vi "nPoints Concept - Servo Motor.vi"() -> ()   [LabVIEW 2014]
uses:
  <vilib>/myRIO/Express VI/Onboard IO/PWM/PWM Express VI.xnode
  <vilib>/myRIO/Instrument Drivers/Onboard IO/PWM/vis/Set Duty Cycle and Frequency.vi
  <vilib>/myRIO/Instrument Drivers/Onboard IO/PWM/PWM.lvlib
  <vilib>/myRIO/Instrument Drivers/Onboard IO/PWM/typedefs/PWM Configuration.ctl
  <vilib>/myRIO/Common/Instrument Driver Framework/myRIO v1.0/PWM/typedefs/PWM Channels Enum.ctl
  <vilib>/myRIO/Common/Instrument Driver Framework/Utilities/typedefs/Generic FPGA Reference.ctl
  <vilib>/myRIO/Common/Instrument Driver Framework/Utilities/typedefs/myRIO v1.0 Reference.ctl
  <vilib>/myRIO/Common/Instrument Driver Framework/Utilities/typedefs/Hardware Version Enum.ctl
  <vilib>/myRIO/Common/Instrument Driver Framework/Utilities/typedefs/myRIO Generic Hardware Reference.ctl
  <vilib>/myRIO/Instrument Drivers/Onboard IO/PWM/typedefs/PWM Reference.ctl
  <vilib>/myRIO/Instrument Drivers/Onboard IO/PWM/vis/myRIO PWM Open.xnode
  <vilib>/myRIO/Common/Instrument Driver Framework/Utilities/vis/Is FPGA Ref Available.vi
  <vilib>/myRIO/Common/Instrument Driver Framework/myRIO v1.0/PWM/vis/myRIO v1.1 Open PWM.vi
  <vilib>/userdefined/High Color/nirio_resource_hc.ctl
panel:
  out "Servo Position":dbl(knob) scale=0.0..180.0
  out "Pulse Time":dbl(slide) scale=0.0..0.002
  out "PWM Signal":waveform(dbl)(graph)
  in  "Stop Button":bool
  in  "PWM Frequency":dbl=50.0 format="%#_g Hz"
  in  "Duty Cycle %":dbl(slide)=0.05 scale=0.05..0.1 scale format="%.3g"
  # "Servo Motor"
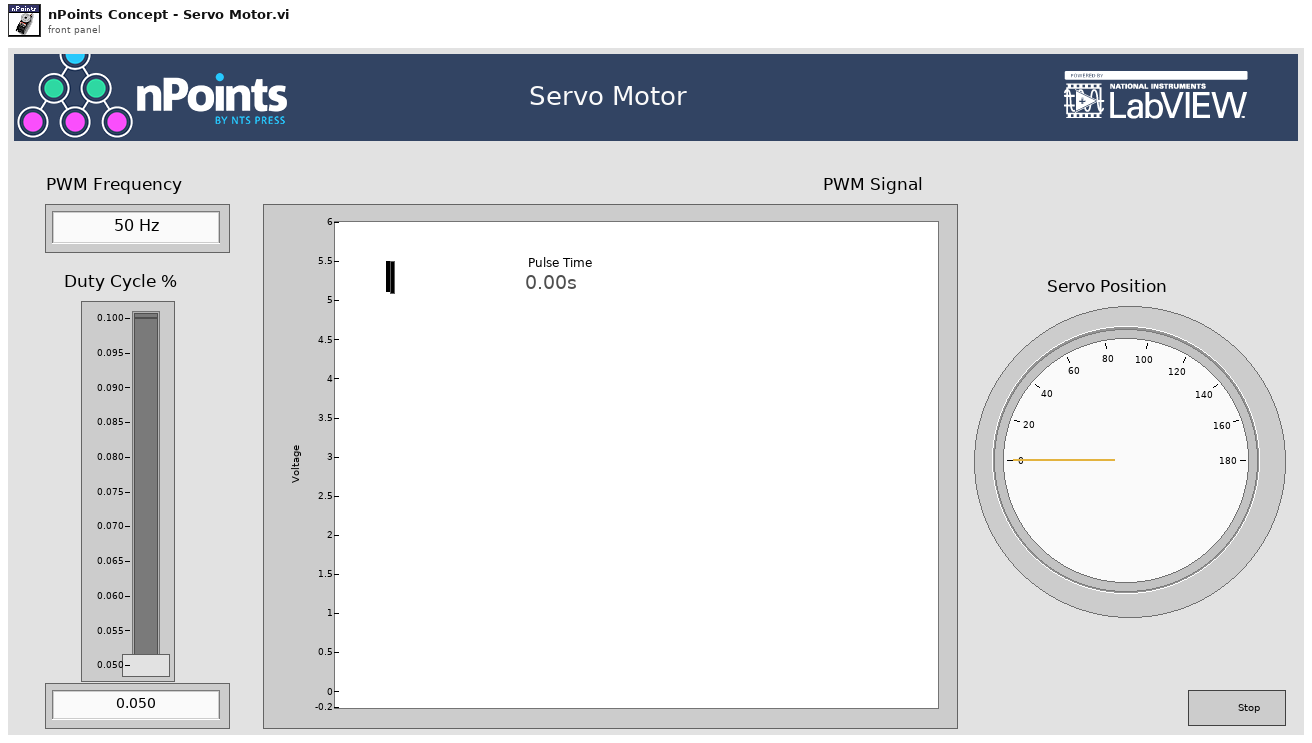
[diagram p1: front panel]
types:
  T1 = typedef "PWM.lvlib/PWM Reference.ctl" = cluster{"myRIO Reference":T2, "PWM Channels Enum":T6, "PWM Configuration":T7}
  T2 = typedef "myRIO Generic Hardware Reference.ctl" = cluster{"myRIO Model":T3, "myRIO Hardware Reference":T4}
  T3 = typedef "Hardware Version Enum.ctl" = enum16{"Unknown", "myRIO-1900", "myRIO-1950"}
  T4 = typedef "myRIO v1.0 Reference.ctl" = cluster{"Generic FPGA Reference":T5, "Allow multiple opens":bool}
  T5 = typedef "Generic FPGA Reference.ctl" = refnum<k20>
  T6 = typedef "PWM Channels Enum.ctl" = enum16{"Not Connected", "C/PWM0", "C/PWM1", "A/PWM0", "A/PWM1", "A/PWM2", "B/PWM0", "B/PWM1", "B/PWM2"}
  T7 = typedef "PWM.lvlib/PWM Configuration.ctl" = cluster{"Frequency":dbl, "Duty Cycle":dbl}
  T8 = typedef "nirio_resource_hc.ctl" = tag
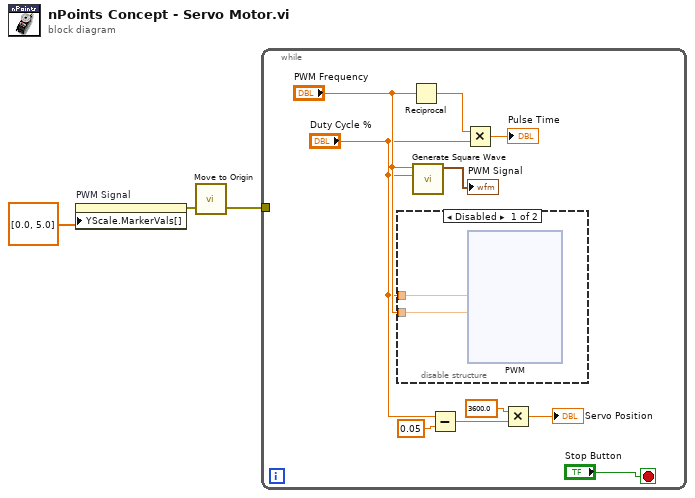
[diagram p0: block diagram]
diagram:
  n1 = property on="PWM Signal" class="WFGraph (strict)"("YScale.MarkerVals[]"=dbl[] [0.0, 5.0] ("Y Scale.Marker Values[]")) -> (error out=w1:errorcluster)  [unwired: 2 in, 1 out]
  n2 = call <userlib>:"Move to Origin.vi"("Error In"=w1) -> ("Error Out"=w3:errorcluster)  [unwired: 2 in]
  n3 = while {
    tunnel: w3 -> [_]
    stop <- "Stop Button" stop-if-true
    n4 = disable-structure shown="Disabled" {
      disable-tunnel: "PWM Frequency" -> [w15 _]
      disable-tunnel: "Duty Cycle %" -> [w14 _]
      frame Disabled {
        n5 = xnode "PWM"("Duty Cycle"=w14, "Frequency [Hz]"=w15) -> ()  [unwired: 1 in, 1 out]
      }
      frame Enabled {
      }
    }
    n6 = Reciprocal(x="PWM Frequency") -> (1/x=w7:dbl)
    n7 = call "Generate Square Wave.vi"("Duty Cycle (%)"="Duty Cycle %", "PWM Frequency"="PWM Frequency") -> ("signal out"=→"PWM Signal":waveform(dbl))  [unwired: 9 in]
    n8 = Subtract(x="Duty Cycle %", y=0.05) -> (x-y=w9:dbl)
    n9 = Multiply(x=w7, y="Duty Cycle %") -> (x*y=→"Pulse Time":dbl)
    n10 = Multiply(x=3600.0 ("y"), y=w9) -> (x*y=→"Servo Position":dbl)
  }
